vi "Split_at_return.vi"(0 "String":string="\r", 1 "offset (0)":i32) -> (2 "before substring":string, 3 "Matched?":bool, 4 "after substring":string, 5 "offset past match":i32)   [LabVIEW 2010]
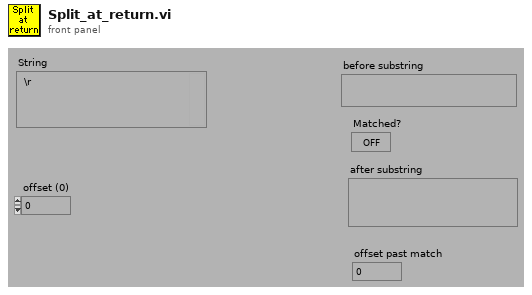
[diagram p1: front panel]
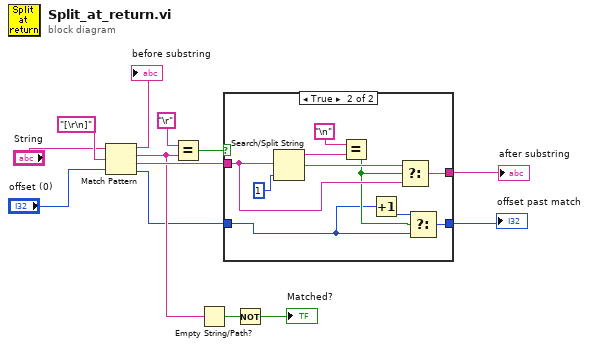
[diagram p0: block diagram]
diagram:
  n1 = Match Pattern(string="String", regular expression="[\r\n]", offset (0)="offset (0)") -> (before substring=→"before substring":string, match substring=w5:string, after substring=w10:string, offset past match=w1:i32)
  n2 = Equal?(x="\r" ("regular expression"), y=w5) -> (x = y?=w11:bool)
  n3 = Empty String/Path?(string/path=w5) -> (empty?=w4:bool)
  n4 = case shown="True" w11 {
    tunnel: w10 -> [w15 w21]
    tunnel: [w15 w20] -> w9
    tunnel: [w14 w16] -> w2
    tunnel: w1 -> [w14 w18]
    frame False {
    }
    frame True {
      n5 = Search/Split String(string=w21, offset (0)=1) -> (substring before match=w22:string, match + rest of string=w23:string)  [unwired: 2 out]
      n6 = Equal?(x="\n" ("regular expression"), y=w22) -> (x = y?=w19:bool)
      n7 = Increment(x=w18) -> (x+1=w17:i32)
      n8 = Select(t=w23, s=w19, f=w21) -> (s? t:f=w20:string)
      n9 = Select(t=w17, s=w19, f=w18) -> (s? t:f=w16:i32)
    }
  }
  "after substring" <- w9
  "offset past match" <- w2
  n10 = Not(x=w4) -> (.not. x?=→"Matched?":bool)
